vi "Get Default Value.vi"(8 "error in":errorcluster, 11 "Object Entry in":refnum<class "Object Entry.lvclass">) -> (0 "error out":errorcluster, 2 "Default Value":string, 3 "Object Entry out":refnum<class "Object Entry.lvclass">)   [LabVIEW 2020, in "CANopen.lvlib" / "Object Entry.lvclass"]
uses:
  Object Entry.lvclass
  Object Entry.lvclass/Object Entry.ctl
  Sub Object/Sub Object.lvclass
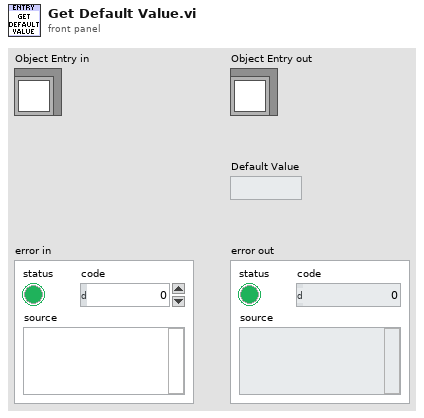
[diagram p1: front panel]
types:
  T1 = typedef "CANopen.lvlib/Object Type.ctl" = u8
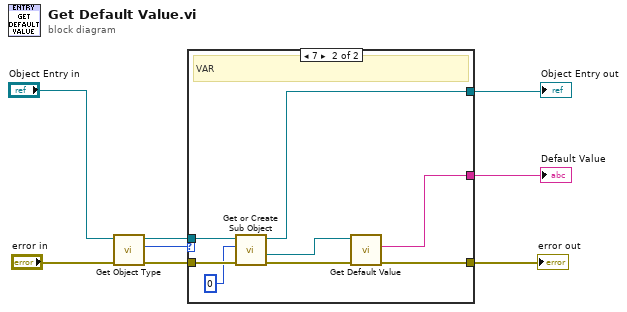
[diagram p0: block diagram]
diagram:
  n1 = call "Get Object Type.vi"("error in"="error in", "Object Entry in"="Object Entry in") -> ("error out"=w3:errorcluster, "Object Type"=w4:T1, "Object Entry out"=w6:refnum<class "Object Entry.lvclass">)  [unwired: 7 in]
  n2 = case shown="7" w4 {
    tunnel: w6 -> [w9 w16]
    tunnel: [w9 w15] -> w5
    tunnel: w3 -> [w10 w18]
    tunnel: [w10 w13] -> w2
    tunnel: [_ w11] -> w1
    frame Default {
    }
    frame 7 {
      # "VAR"
      n3 = call "Get or Create Sub Object.vi"("error in"=w18, "Sub Index"=u8 0, "Obj Entry in"=w16) -> ("error out"=w17:errorcluster, "Sub Object"=w12:refnum<class "Sub Object.lvclass">, "Obj Entry out"=w15:refnum<class "Object Entry.lvclass">)  [unwired: 6 in]
      n4 = call "Get Default Value.vi"("error in"=w17, "Sub Object in"=w12) -> ("error out"=w13:errorcluster, "Default Value"=w11:string)  [unwired: 7 in, 1 out]
    }
  }
  "error out" <- w2
  "Object Entry out" <- w5
  "Default Value" <- w1
